vi "Edit Expression.vi"(8 "Coords":T2, 11 "Expr In":string) -> (3 "Expr Out":string)   [LabVIEW 2020, in "Trigger.xctl"]
uses:
  Trigger.xctl
  <vilib>/Utility/miscctls.llb/LVPoint32TypeDef.ctl
  epl-vi-lib/Utility VIs/Error Handling VIs/Error-Library Action.ctl
panel:
  in  "Tab Control":enum32{"Hist", "Error"}(tab)
  out "histogram":T1(graph)
  out "X-axis":dbl(slide) scale=850.0..4150.0
  out "Message":string
  out "replot":bool
  in  "Expr":string
  in  "Cancel":bool
  in  "OK":bool
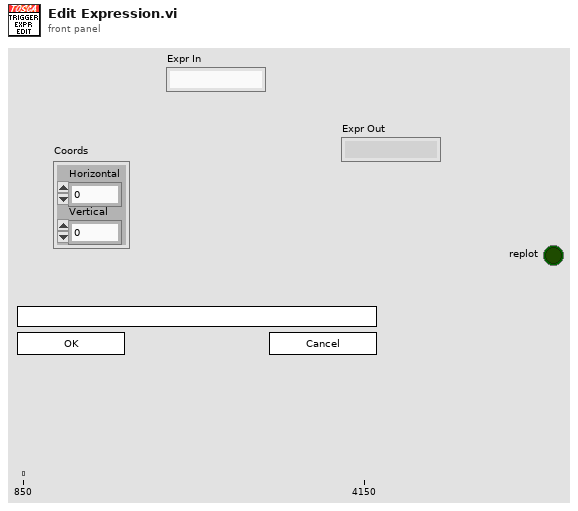
[diagram p1: front panel]
types:
  T1 = cluster{"X Values":dbl[], "Histogram: h(x)":dbl[]}[]
  T2 = typedef "LVPoint32TypeDef.ctl" = cluster{"Horizontal":i32, "Vertical":i32}
  T3 = typedef "Error-Library Action.ctl" = enum16{"NONE", "Register", "Read"}
  T4 = typedef "Error Description.ctl" = cluster{"Code":i32, "Description":string, "Details":string}
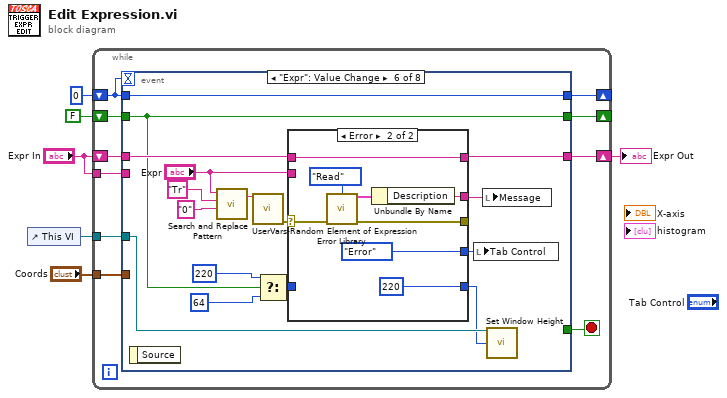
[diagram p0: block diagram]
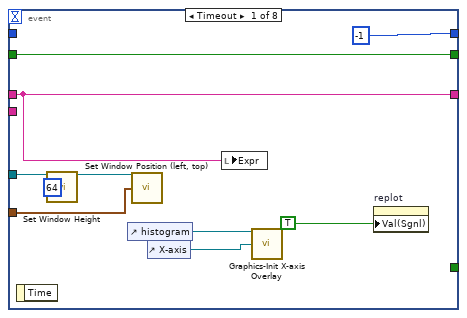
[diagram p2: hidden frame]
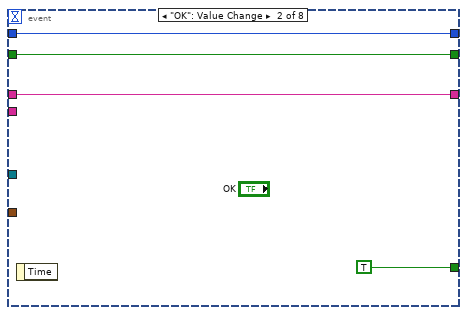
[diagram p3: hidden frame]
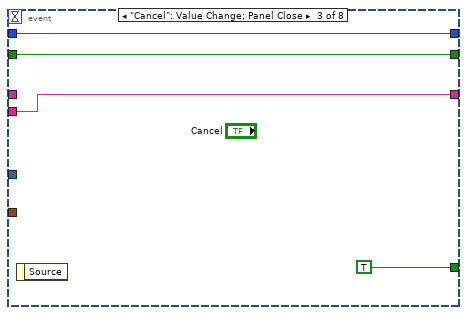
[diagram p4: hidden frame]
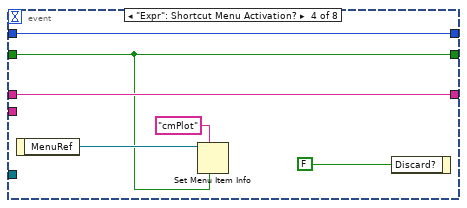
[diagram p5: hidden frame]
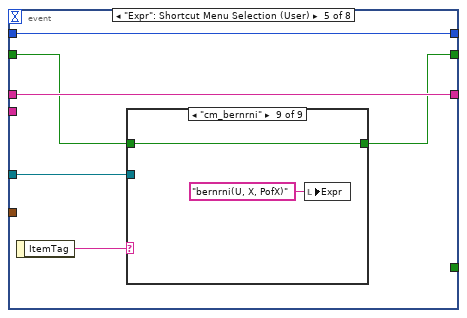
[diagram p6: hidden frame]
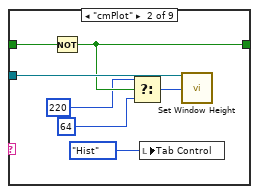
[diagram p8: hidden frame]
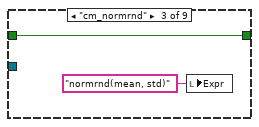
[diagram p9: hidden frame]
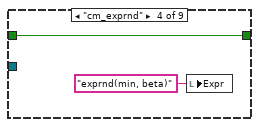
[diagram p10: hidden frame]
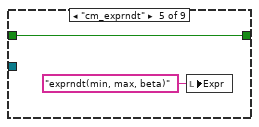
[diagram p11: hidden frame]
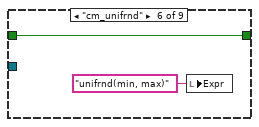
[diagram p12: hidden frame]
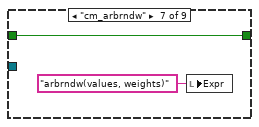
[diagram p13: hidden frame]
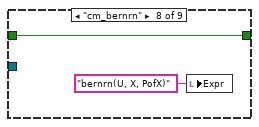
[diagram p14: hidden frame]
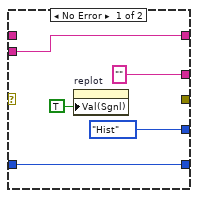
[diagram p15: hidden frame]
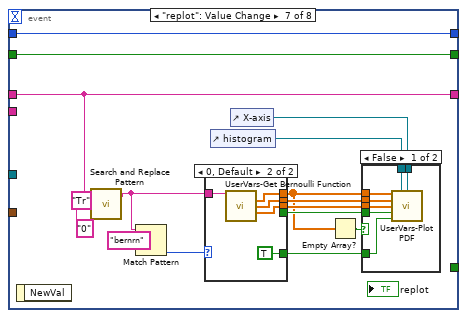
[diagram p16: hidden frame]
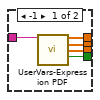
[diagram p17: hidden frame]
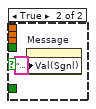
[diagram p18: hidden frame]
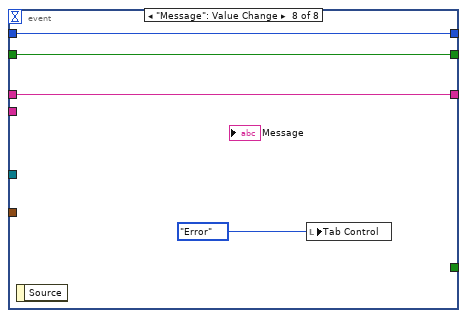
[diagram p19: hidden frame]
diagram:
  n1 = control-ref of="This VI"() -> (w2:refnum<vi>)
  n2 = while {
    shift-right: [w15] -> w6
    shift-left: "Expr In" -> [w16]
    shift-right: [w13] -> _
    shift-left: 0 -> [w12]
    tunnel: "Expr In" -> [w11]
    tunnel: "Coords" -> [w10]
    tunnel: w2 -> [w9]
    shift-right: [w7] -> _
    shift-left: FALSE -> [w8]
    stop <- w14 stop-if-true
    n3 = event shown="[5] \"Expr\": Value Change" {
      selector: _ -> [_ _ _ _ _ _ _ _]
      dyn-events: _ -> [_ _ _ _ _ _ _ _]
      timeout: w12 -> [_ _ _ _ _ _ _ _]
      tunnel: w16 -> [w25 w28 _ w40 w46 w82 w102 w135]
      tunnel: [w25 w28 w32 w40 w46 w81 w102 w135] -> w15
      tunnel: [_ TRUE TRUE _ _ _ _ _] -> w14
      tunnel: w12 -> [_ w29 w33 w39 w45 w84 w113 w134]
      tunnel: [-1 w29 w33 w39 w45 w84 w113 w134] -> w13
      tunnel: w11 -> [_ _ w32 _ _ _ _ _]
      tunnel: w10 -> [w24 _ _ _ _ _ _ _]
      tunnel: w9 -> [w19 _ _ _ w43 w79 _ _]
      tunnel: w8 -> [w20 w27 w31 w36 w44 w75 w111 w133]
      tunnel: [w20 w27 w31 w36 w42 w75 w111 w133] -> w7
      event Timeout {
        n4 = event-data() -> ()  [unwired: 1 in, 1 out]
        n5 = call "Set Window Height.vi"("VI in"=w19, "Height"=i16 64) -> ("VI out"=w18:refnum<vi>)  [unwired: 12 in, 1 out]
        n6 = control-ref of="histogram"() -> (w23:refnum<vi>)
        n7 = call "Set Window Position (left, top).vi"("VI in"=w18, "Coords"=w24) -> ()  [unwired: 12 in, 2 out]
        n8 = control-ref of="X-axis"() -> (w22:refnum<vi>)
        n9 = local write "Expr"(w25) -> ()
        n10 = call "Graphics-Init X-axis Overlay.vi"("Ctl Refnum"=w23, "X-axis slider"=w22) -> ()  [unwired: 13 in, 1 out]
        n11 = property on="replot" class="Bool (strict)"("Val(Sgnl)"=TRUE ("Value (Signaling)")) -> ()  [unwired: 2 in, 2 out]
      }
      event "OK": Value Change {
        n12 = event-data() -> ()  [unwired: 1 in, 1 out]
      }
      event "Cancel": Value Change; Panel Close {
        n13 = event-data() -> ()  [unwired: 1 in, 1 out]
      }
      event "Expr": Shortcut Menu Activation? {
        n14 = event-data() -> ("MenuRef"=w38:refnum<k9>)  [unwired: 1 in]
        n15 = Set Menu Item Info(6:w36, 7:"cmPlot" ("item tag"), 11:w38) -> ()  [unwired: 4 in, 2 out]
        n16 = event-data("Discard?"=FALSE) -> ()  [unwired: 1 in, 1 out]
      }
      event "Expr": Shortcut Menu Selection (User) {
        n17 = event-data() -> ("ItemTag"=w41:string)  [unwired: 1 in]
        n18 = case shown="\"cm_bernrni\"" w41 {
          tunnel: w44 -> [w47 w54 w56 w58 w60 w62 w64 w66 w68]
          tunnel: w43 -> [_ w53 _ _ _ _ _ _ _]
          tunnel: [w47 w52 w56 w58 w60 w62 w64 w66 w68] -> w42
          frame "False", Default {
          }
          frame "cmPlot" {
            n19 = Not(x=w54) -> (.not. x?=w52:bool)
            n20 = Select(t=i16 220 ("Height"), s=w52, f=i16 64 ("Height")) -> (s? t:f=w51:i16)
            n21 = local write "Tab Control"(enum32{"Hist", "Error"}."Hist" ("Tab Control")) -> ()
            n22 = call "Set Window Height.vi"("VI in"=w53, "Height"=w51) -> ()  [unwired: 12 in, 2 out]
          }
          frame "cm_normrnd" {
            n23 = local write "Expr"("normrnd(mean, std)" ("Expr")) -> ()
          }
          frame "cm_exprnd" {
            n24 = local write "Expr"("exprnd(min, beta)" ("Expr")) -> ()
          }
          frame "cm_exprndt" {
            n25 = local write "Expr"("exprndt(min, max, beta)" ("Expr")) -> ()
          }
          frame "cm_unifrnd" {
            n26 = local write "Expr"("unifrnd(min, max)" ("Expr")) -> ()
          }
          frame "cm_arbrndw" {
            n27 = local write "Expr"("arbrndw(values, weights)" ("Expr")) -> ()
          }
          frame "cm_bernrn" {
            n28 = local write "Expr"("bernrn(U, X, PofX)" ("Expr")) -> ()
          }
          frame "cm_bernrni" {
            n29 = local write "Expr"("bernrni(U, X, PofX)" ("Expr")) -> ()
          }
        }
      }
      event "Expr": Value Change {
        n30 = event-data() -> ()  [unwired: 1 in, 1 out]
        n31 = call <vilib>:"Search and Replace Pattern.vi"("string"="Expr", "regular expression (\"\")"="Tr" ("regular expression (\"\")"), "replace string (\"\")"="0" ("replace string (\"\")")) -> ("result string"=w70:string)  [unwired: 2 in, 1 out]
        n32 = call "UserVars-Random Element of Expression.vi"("Expr"=w70) -> ("error out"=w83:errorcluster)  [unwired: 12 in, 2 out]
        n33 = Select(t=i16 220 ("Height"), s=w75, f=i16 64 ("Height")) -> (s? t:f=w74:i16)
        n34 = case shown="Error" w83 {
          selector: w83 -> [_ w96]
          tunnel: w82 -> [_ w97]
          tunnel: [w85 w97] -> w81
          tunnel: "Expr" -> [w85 _]
          tunnel: ["" ("Description") w90] -> w73
          tunnel: [_ w94] -> _
          tunnel: [enum32{"Hist", "Error"}."Hist" ("Tab Control") enum32{"Hist", "Error"}."Error" ("Tab Control")] -> w80
          tunnel: [w86 i16 220 ("Height")] -> w78
          tunnel: w74 -> [w86 _]
          frame No Error {
            n35 = property on="replot" class="Bool (strict)"("Val(Sgnl)"=TRUE ("Value (Signaling)")) -> ()  [unwired: 2 in, 2 out]
          }
          frame Error {
            n36 = call "Error Library.vi"("action"=Error-Library_Action."Read", "error in"=w96) -> ("Entry"=w95:T4, "error thru"=w94:errorcluster)  [unwired: 11 in, 1 out]
            n37 = Unbundle By Name(w95) -> ("Description"=w90:string)
          }
        }
        n38 = local write "Tab Control"(w80) -> ()
        n39 = local write "Message"(w73) -> ()
        n40 = call "Set Window Height.vi"("VI in"=w79, "Height"=w78) -> ()  [unwired: 12 in, 2 out]
      }
      event "replot": Value Change {
        n41 = event-data() -> ()  [unwired: 1 in, 1 out]
        n42 = call <vilib>:"Search and Replace Pattern.vi"("string"=w102, "regular expression (\"\")"="Tr" ("regular expression (\"\")"), "replace string (\"\")"="0" ("replace string (\"\")")) -> ("result string"=w101:string)  [unwired: 2 in, 1 out]
        n43 = Match Pattern(string=w101, regular expression="bernrn") -> (offset past match=w99:i32)  [unwired: 1 in, 3 out]
        n44 = case shown="0, Default" w99 {
          tunnel: [w118 w120] -> w109
          tunnel: [w117 w119] -> w108
          tunnel: [w116 _] -> w107
          tunnel: [w115 w121] -> w106
          tunnel: w101 -> [w114 w122]
          tunnel: [_ TRUE] -> w98
          frame -1 {
            n45 = call "UserVars-Expression PDF.vi"("Expr"=w114) -> ("X"=w115:dbl[], "PDF"=w118:dbl[], "refpts"=w117:dbl[], "mass function"=w116:bool)  [unwired: 10 in, 1 out]
          }
          frame 0, Default {
            n46 = call "UserVars-Get Bernoulli Function.vi"("Expr in"=w122) -> ("X"=w121:dbl[], "PDF"=w120:dbl[], "Ref Pts"=w119:dbl[])  [unwired: 11 in, 1 out]
          }
        }
        n47 = control-ref of="histogram"() -> (w110:refnum<vi>)
        n48 = control-ref of="X-axis"() -> (w112:refnum<vi>)
        n49 = Empty Array?(array=w106) -> (empty?=w105:bool)
        n50 = case shown="False" w105 {
          tunnel: w112 -> [w130 _]
          tunnel: w110 -> [w129 _]
          tunnel: w106 -> [w128 _]
          tunnel: w109 -> [w127 _]
          tunnel: w108 -> [w126 _]
          tunnel: w107 -> [w125 _]
          tunnel: w98 -> [w124 _]
          frame False {
            n51 = call "UserVars-Plot PDF.vi"("X"=w128, "XYGraph"=w129, "X-axis"=w130, "PDF"=w127, "refpts"=w126, "mass"=w125, "bernoulli"=w124) -> ()  [unwired: 9 in]
          }
          frame True {
            n52 = property on="Message" class="Str"("Val(Sgnl)"="Distribution too complicated to display." ("Value (Signaling)")) -> ()  [unwired: 2 in, 2 out]
          }
        }
      }
      event "Message": Value Change {
        n53 = event-data() -> ()  [unwired: 1 in, 1 out]
        n54 = local write "Tab Control"(enum32{"Hist", "Error"}."Error" ("Tab Control")) -> ()
      }
    }
  }
  "Expr Out" <- w6
